vi "spot size 2D.vi"(7 "Threshold for 2nd mom":dbl=0.05 format="%#_13g", 8 "error in (no error)":errorcluster, 9 "X Centroid":sgl, 10 "Y Centroid":sgl, 11 "Refnum in":T1) -> (0 "w0y via 2nd mom":sgl, 1 "w0x via 2nd mom":sgl, 2 "FWHMx (pix)":dbl, 3 "FWHMy (pix)":dbl, 4 "error out":errorcluster)   [LabVIEW 2013]
uses:
  <vilib>/vision/Image Controls.llb/IMAQ Image.ctl
  <vilib>/vision/NI_Vision_Development_Module.lvlib
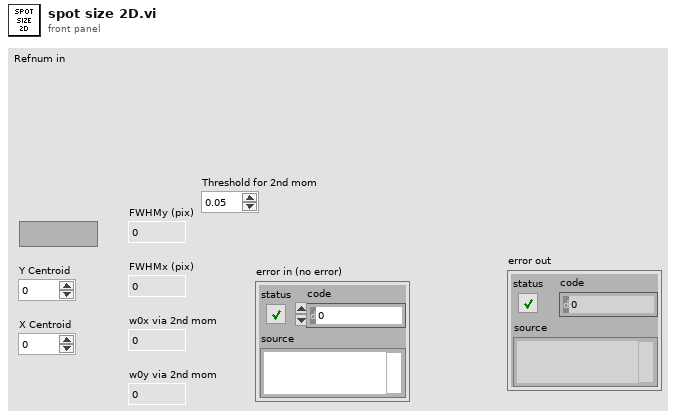
[diagram p1: front panel]
types:
  T1 = typedef "IMAQ Image.ctl" = refnum<image>
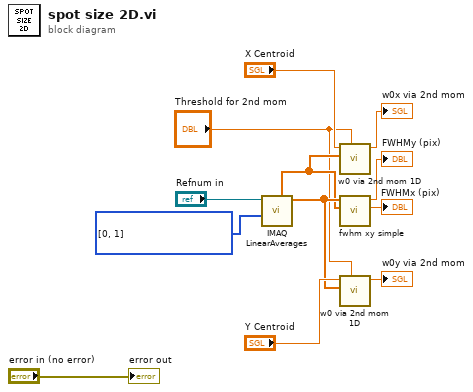
[diagram p0: block diagram]
diagram:
  w5 = i32[] [0, 1] items=["X Axis Averages", "Y Axis Averages", "X + Y Axis Averages", "X - Y Axis Averages"] ("Averages")
  n1 = call "IMAQ LinearAverages"("Averages"=w5, "Image Src"="Refnum in") -> ("Y Axis Averages"=w7:sgl[], "X Axis Averages"=w6:sgl[])  [unwired: 2 in, 6 out]
  n2 = call "w0 via 2nd mom 1D.vi"("Threshold for 2nd mom"="Threshold for 2nd mom", "Input array"=w6, "Centroid"="X Centroid") -> ("w0 via 2nd mom"=→"w0x via 2nd mom":sgl)  [unwired: 8 in]
  n3 = call "fwhm xy simple.vi"("X Axis Averages"=w6, "Y Axis Averages"=w7) -> ("FWHM (pix) 2"=→"FWHMx (pix)":dbl, "FWHM (pix)"=→"FWHMy (pix)":dbl)  [unwired: 8 in]
  n4 = call "w0 via 2nd mom 1D.vi"("Threshold for 2nd mom"="Threshold for 2nd mom", "Input array"=w7, "Centroid"="Y Centroid") -> ("w0 via 2nd mom"=→"w0y via 2nd mom":sgl)  [unwired: 8 in]
  "error out" <- "error in (no error)"
